vi "4000_tx_rx_(chksum).vi"(3 "Port Name":string, 4 "Channel Name":string, 5 "Write String":string="#FC") -> (0 "Comment out":string, 1 "millisecond timer value":u32, 2 "Read":string=">+00.000")   [LabVIEW 2010]
panel:
  in  "?":bool=TRUE
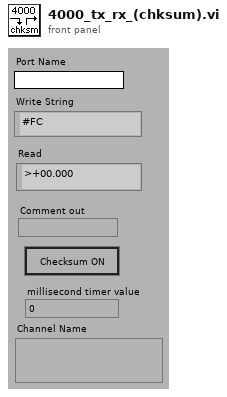
[diagram p1: front panel]
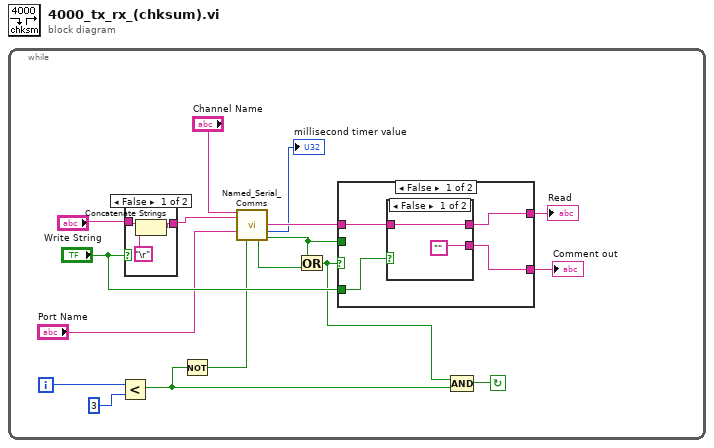
[diagram p0: block diagram]
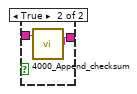
[diagram p2: hidden frame]
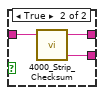
[diagram p3: hidden frame]
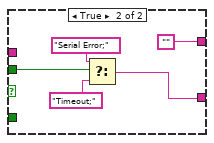
[diagram p4: hidden frame]
diagram:
  n1 = while {
    i -> [w3]
    stop <- w5 continue-if-true
    n2 = Less?(x=w3, y=3) -> (x < y?=w2:bool)
    n3 = case shown="False" "?" {
      tunnel: [w19 w22] -> w8
      tunnel: "Write String" -> [w20 w21]
      frame False {
        n4 = Concatenate Strings(w20, "\r") -> (w19:string)
      }
      frame True {
        n5 = call "4000_Append_checksum.vi"("ADAM command"=w21) -> ("ADAM string to send"=w22:string)
      }
    }
    n6 = Not(x=w2) -> (.not. x?=w1:bool)
    n7 = call "Named_Serial_Comms.vi"("Channel Name"="Channel Name", "Write String"=w8, "Port Name"="Port Name", "Log Errors?"=w1) -> ("Read"=w16:string, "millisecond timer value"=→"millisecond timer value":u32, "Timed out"=w13:bool, "Serial Error"=w12:bool)  [unwired: 5 in, 3 out]
    n8 = Or(x=w12, y=w13) -> (x .or. y?=w4:bool)
    n9 = case shown="False" w4 {
      tunnel: w16 -> [w26 _]
      tunnel: [w25 w35] -> w15
      tunnel: [w24 ""] -> w14
      tunnel: w12 -> [_ w36]
      tunnel: "?" -> [w23 _]
      frame False {
        n10 = case shown="False" w23 {
          tunnel: w26 -> [w28 w31]
          tunnel: ["" w30] -> w25
          tunnel: [w28 w29] -> w24
          frame False {
          }
          frame True {
            n11 = call "4000_Strip_Checksum.vi"("ADAM response"=w31) -> ("Comment out"=w30:string, "ADAM reading"=w29:string)  [unwired: 3 out]
          }
        }
      }
      frame True {
        n12 = Select(t="Serial Error;", s=w36, f="Timeout;") -> (s? t:f=w35:string)
      }
    }
    "Read" <- w14
    "Comment out" <- w15
    n13 = Compound Arithmetic op=AND(w4, w2) -> (w5:bool)
  }
